vi "subVI_XPID.vi"(8 "Cumulative Error In":dbl, 9 "Previous Error":dbl, 10 "Encoder Position [mm]":dbl, 11 "Desired Position [mm]":dbl) -> (0 "Cumulative Error Out":dbl, 1 "Error":dbl, 3 "Control Signal [V]":dbl)   [LabVIEW 2019]
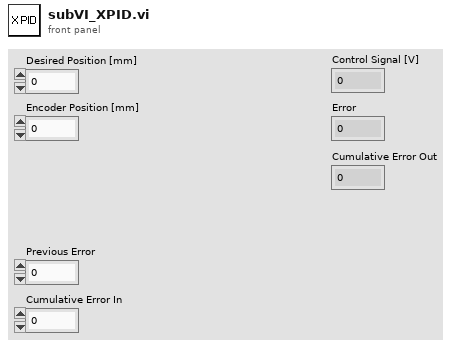
[diagram p1: front panel]
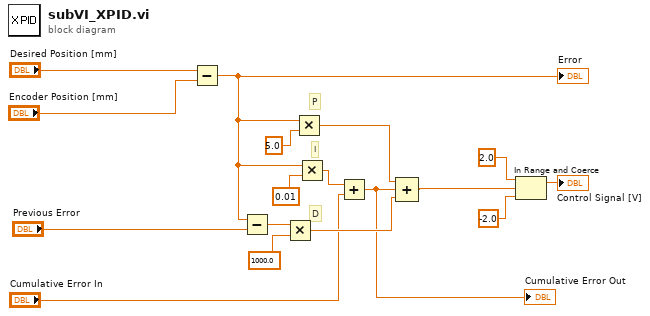
[diagram p0: block diagram]
diagram:
  # "D"
  # "I"
  # "P"
  n1 = Subtract(x="Desired Position [mm]", y="Encoder Position [mm]") -> (x-y=w1:dbl)
  "Error" <- w1
  n2 = Subtract(x=w1, y="Previous Error") -> (x-y=w14:dbl)
  n3 = Multiply(x=w14, y=1000.0) -> (x*y=w12:dbl)
  n4 = Multiply(x=w1, y=5.0) -> (x*y=w13:dbl)
  n5 = Multiply(x=w1, y=0.01) -> (x*y=w10:dbl)
  n6 = Add(x=w10, y="Cumulative Error In") -> (x+y=w6:dbl)
  "Cumulative Error Out" <- w6
  n7 = Compound Arithmetic op=ADD(w13, w6, w12) -> (w2:dbl)
  n8 = In Range and Coerce(upper limit=2.0, x=w2, lower limit=-2.0) -> (coerced(x)=→"Control Signal [V]":dbl)  [unwired: 1 out]
